vi "Fulltrackasbackground_171213.vi"(10 "FullTracakonSegments":picture, 11 "FullTrackonNormalMouseBackground":picture) -> ()   [LabVIEW 2016]
uses:
  Globaltracker.vi
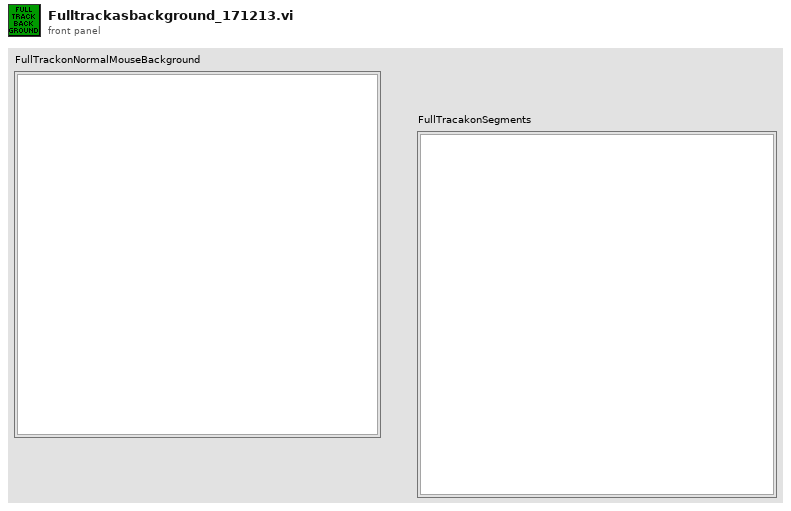
[diagram p1: front panel]
types:
  T1 = cluster{"left":i16, "top":i16, "right":i16, "bottom":i16}
  T2 = typedef "imagedata.ctl" = cluster{"image type":i32, "image depth":i32, "image":u8[], "mask":u8[], "colors":u32[], "Rectangle":cluster{"left":i16, "top":i16, "right":i16, "bottom":i16}}
  T3 = cluster{"image type":i32, "image depth":i32, "image":u8[], "mask":u8[], "colors":u32[], cluster{i32, i32, i32, i32}}
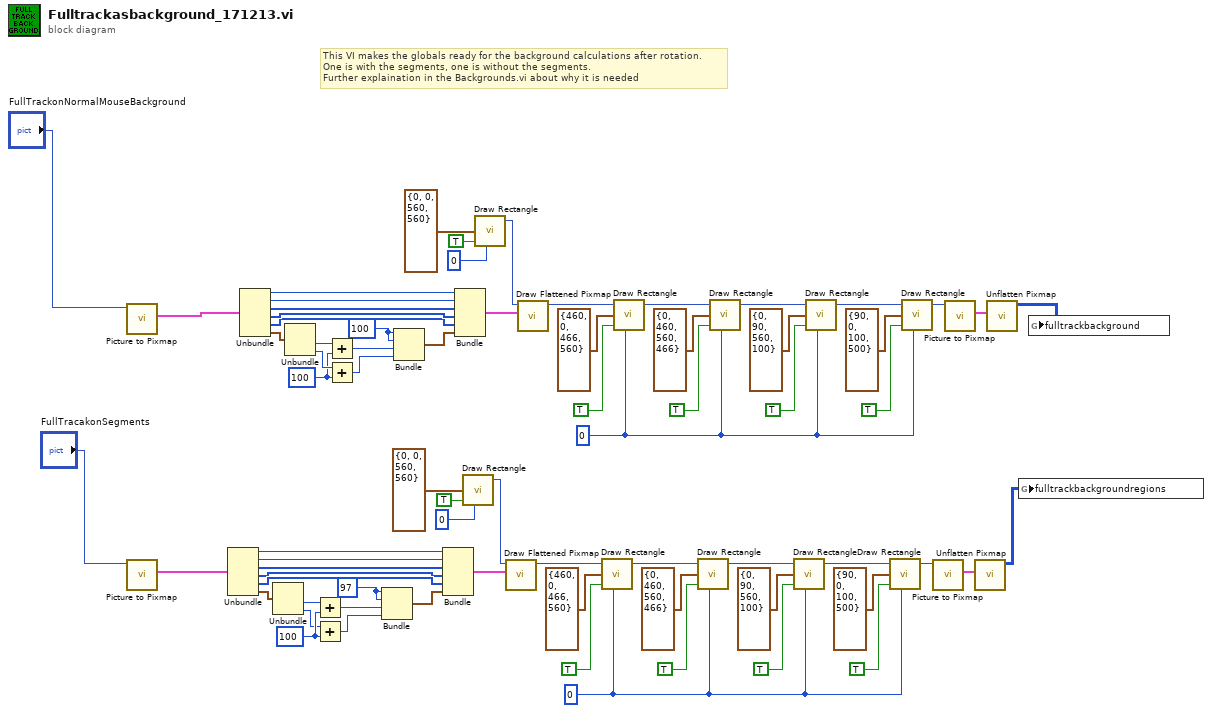
[diagram p0: block diagram]
diagram:
  w29 = 100
  w36 = 0
  w11 = 97
  w48 = 100
  w41 = 0
  w67 = 100
  # "This VI makes the globals ready for the background calculations after rotation.\nOne is with the segments, one is without the segments. \nFurther explaination in the Backgrounds.vi about why it is needed"
  n1 = call <vilib>:"Picture to Pixmap.vi"("picture"="FullTrackonNormalMouseBackground") -> ("image data"=w1:T2)  [unwired: 9 in, 1 out]
  n2 = call <vilib>:"Picture to Pixmap.vi"("picture"="FullTracakonSegments") -> ("image data"=w7:T2)  [unwired: 9 in, 1 out]
  n3 = Unbundle(w7) -> ("image type"=w14:i32, "image depth"=w15:i32, "image"=w16:u8[], "mask"=w17:u8[], "colors"=w18:u32[], "Rectangle"=w8:T1)
  n4 = Unbundle(w1) -> ("image type"=w64:i32, "image depth"=w63:i32, "image"=w62:u8[], "mask"=w61:u8[], "colors"=w60:u32[], "Rectangle"=w70:T1)
  n5 = Unbundle(w8) -> ("right"=w9:i16, "bottom"=w10:i16)  [unwired: 2 out]
  n6 = Unbundle(w70) -> ("right"=w69:i16, "bottom"=w68:i16)  [unwired: 2 out]
  n7 = Add(x=w9, y=w29) -> (x+y=w12:i32)
  n8 = Add(x=w10, y=w29) -> (x+y=w13:i32)
  n9 = Add(x=w69, y=w48) -> (x+y=w66:i32)
  n10 = Add(x=w68, y=w48) -> (x+y=w65:i32)
  n11 = Bundle(w11, w11, w12, w13) -> (w19:cluster{i32, i32, i32, i32})  [unwired: 1 in]
  n12 = Bundle(w67, w67, w66, w65) -> (w59:cluster{i32, i32, i32, i32})  [unwired: 1 in]
  n13 = Bundle("image type"=w14, "image depth"=w15, "image"=w16, "mask"=w17, "colors"=w18, w19) -> (w20:T3)  [unwired: 1 in]
  n14 = Bundle("image type"=w64, "image depth"=w63, "image"=w62, "mask"=w61, "colors"=w60, w59) -> (w58:T3)  [unwired: 1 in]
  n15 = call <vilib>:"Draw Rectangle.vi"("rect"=T1 {"left"=0, "top"=0, "right"=560, "bottom"=560}, "fill?(F)"=TRUE, "color(black)"=0) -> ("new picture"=w21:picture)  [unwired: 6 in]
  n16 = call <vilib>:"Draw Rectangle.vi"("rect"=T1 {"left"=0, "top"=0, "right"=560, "bottom"=560}, "fill?(F)"=TRUE, "color(black)"=0) -> ("new picture"=w57:picture)  [unwired: 6 in]
  n17 = call <vilib>:"Draw Flattened Pixmap.vi"("image data"=w20, "picture"=w21) -> ("new picture"=w24:picture)  [unwired: 7 in]
  n18 = call <vilib>:"Draw Flattened Pixmap.vi"("image data"=w58, "picture"=w57) -> ("new picture"=w54:picture)  [unwired: 7 in]
  n19 = call <vilib>:"Draw Rectangle.vi"("picture"=w24, "rect"=T1 {"left"=460, "top"=0, "right"=466, "bottom"=560}, "fill?(F)"=TRUE, "color(black)"=w36) -> ("new picture"=w28:picture)  [unwired: 5 in]
  n20 = call <vilib>:"Draw Rectangle.vi"("picture"=w54, "rect"=T1 {"left"=460, "top"=0, "right"=466, "bottom"=560}, "fill?(F)"=TRUE, "color(black)"=w41) -> ("new picture"=w50:picture)  [unwired: 5 in]
  n21 = call <vilib>:"Draw Rectangle.vi"("picture"=w28, "rect"=T1 {"left"=0, "top"=460, "right"=560, "bottom"=466}, "fill?(F)"=TRUE, "color(black)"=w36) -> ("new picture"=w32:picture)  [unwired: 5 in]
  n22 = call <vilib>:"Draw Rectangle.vi"("picture"=w50, "rect"=T1 {"left"=0, "top"=460, "right"=560, "bottom"=466}, "fill?(F)"=TRUE, "color(black)"=w41) -> ("new picture"=w45:picture)  [unwired: 5 in]
  n23 = call <vilib>:"Draw Rectangle.vi"("picture"=w32, "rect"=T1 {"left"=0, "top"=90, "right"=560, "bottom"=100}, "fill?(F)"=TRUE, "color(black)"=w36) -> ("new picture"=w35:picture)  [unwired: 5 in]
  n24 = call <vilib>:"Draw Rectangle.vi"("picture"=w45, "rect"=T1 {"left"=0, "top"=90, "right"=560, "bottom"=100}, "fill?(F)"=TRUE, "color(black)"=w41) -> ("new picture"=w42:picture)  [unwired: 5 in]
  n25 = call <vilib>:"Draw Rectangle.vi"("picture"=w35, "rect"=T1 {"left"=90, "top"=0, "right"=100, "bottom"=500}, "fill?(F)"=TRUE, "color(black)"=w36) -> ("new picture"=w38:picture)  [unwired: 5 in]
  n26 = call <vilib>:"Draw Rectangle.vi"("picture"=w42, "rect"=T1 {"left"=90, "top"=0, "right"=100, "bottom"=500}, "fill?(F)"=TRUE, "color(black)"=w41) -> ("new picture"=w39:picture)  [unwired: 5 in]
  n27 = call <vilib>:"Picture to Pixmap.vi"("picture"=w38) -> ("image data"=w37:T2)  [unwired: 9 in, 1 out]
  n28 = call <vilib>:"Picture to Pixmap.vi"("picture"=w39) -> ("image data"=w40:T2)  [unwired: 9 in, 1 out]
  n29 = call <vilib>:"Unflatten Pixmap.vi"("image data"=w37) -> ("24-bit pixmap"=w3:u32[][])  [unwired: 4 in, 6 out]
  n30 = call <vilib>:"Unflatten Pixmap.vi"("image data"=w40) -> ("24-bit pixmap"=w2:u32[][])  [unwired: 4 in, 6 out]
  n31 = global write "Globaltracker.vi" "fulltrackbackgroundregions"(w3) -> ()
  n32 = global write "Globaltracker.vi" "fulltrackbackground"(w2) -> ()
